vi "Get UI Ref.vi"(8 "error in (no error)":errorcluster, 11 "9402 in":refnum<class "9402.lvclass">) -> (0 "error out":errorcluster, 1 "Show SubPanel?":bool, 2 "VI Refnum":refnum<vi>, 3 "9402 out":refnum<class "9402.lvclass">)   [LabVIEW 2017, in "Modules.lvlib" / "9402.lvclass"]
uses:
  9402.lvclass
  C:/Users/dbuck/Documents/GitHub/Scan-Engine-Custom-Device-Classes/Source/RSI Module/RSI Module.lvclass
  SD Module/SD Module.lvclass
  RSI Module/RSI Module.lvclass
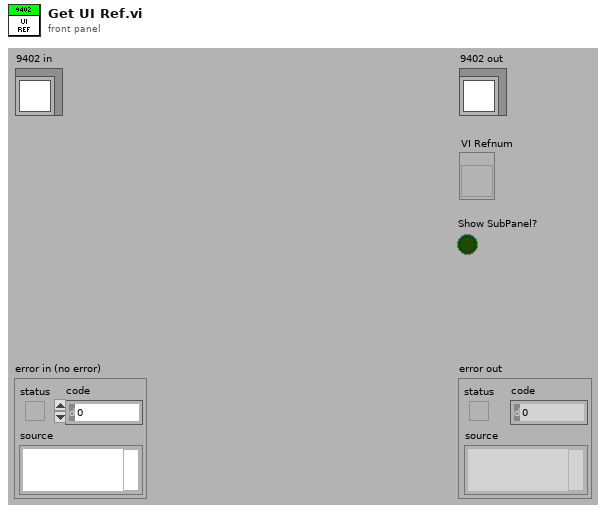
[diagram p1: front panel]
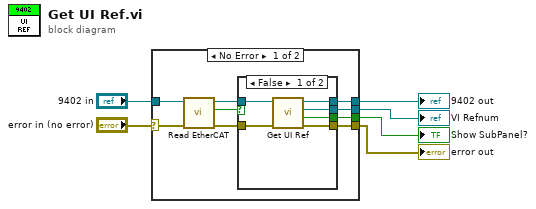
[diagram p0: block diagram]
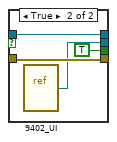
[diagram p2: hidden frame]
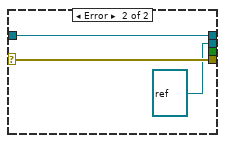
[diagram p3: hidden frame]
diagram:
  n1 = case shown="No Error" "error in (no error)" {
    selector: "error in (no error)" -> [w12 w28]
    tunnel: [w7 w28] -> w1
    tunnel: [w9 w27] -> w4
    tunnel: "9402 in" -> [w13 w27]
    tunnel: [w15 refnum<vi> refnum] -> w3
    tunnel: [w14 _] -> w2
    frame No Error {
      n2 = call "Read EtherCAT.vi"("error in (no error)"=w12, "RSI Module in"=w13) -> ("error out"=w8:errorcluster, "EtherCAT?"=w11:bool, "RSI Module out"=w10:refnum<class "9402.lvclass">)  [unwired: 7 in]
      n3 = case shown="False" w11 {
        tunnel: [w21 w22] -> w15
        tunnel: [w20 TRUE] -> w14
        tunnel: w10 -> [w19 w23]
        tunnel: [w18 w23] -> w9
        tunnel: w8 -> [w17 w24]
        tunnel: [w16 w24] -> w7
        frame False {
          n4 = call-parent "Get UI Ref.vi"("error in (no error)"=w17, "SD Module in"=w19) -> ("error out"=w16:errorcluster, "Show SubPanel?"=w20:bool, "VI Refnum"=w21:refnum<vi>, "SD Module out"=w18:refnum<class "9402.lvclass">)  [unwired: 6 in]
        }
        frame True {
          n5 = vi-ref "9402_UI.vi"() -> (w22:refnum<vi>)
        }
      }
    }
    frame Error {
    }
  }
  "error out" <- w1
  "9402 out" <- w4
  "VI Refnum" <- w3
  "Show SubPanel?" <- w2
